vi "get_version_numbering.vi"(11 "local version in":string) -> (0 "resulting string":string, 1 "revision out":i32, 2 "minor out":i32, 3 "mayor out":i32)   [LabVIEW 2010, in "HelioUpdateMH100803.lvclass"]
uses:
  HelioUpdateMH100803.lvclass
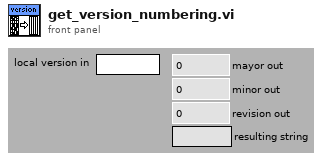
[diagram p1: front panel]
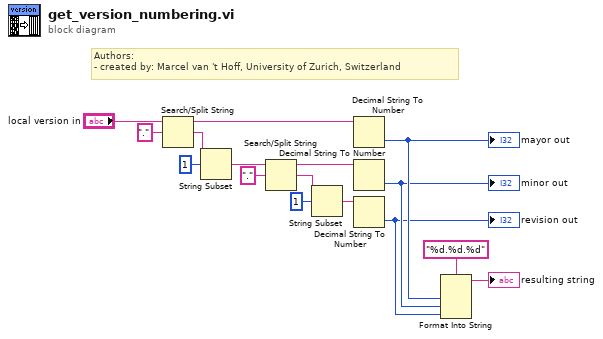
[diagram p0: block diagram]
diagram:
  # "Authors: \n- created by: Marcel van 't Hoff, University of Zurich, Switzerland"
  n1 = Search/Split String(string="local version in", search string/char (-)=".") -> (substring before match=w9:string, match + rest of string=w10:string)  [unwired: 1 in, 1 out]
  n2 = String Subset(string=w10, offset (0)=1) -> (substring=w11:string)  [unwired: 1 in]
  n3 = Search/Split String(string=w11, search string/char (-)=".") -> (substring before match=w15:string, match + rest of string=w13:string)  [unwired: 1 in, 1 out]
  n4 = String Subset(string=w13, offset (0)=1) -> (substring=w16:string)  [unwired: 1 in]
  n5 = Decimal String To Number(string=w9) -> (number=w5:i32)  [unwired: 2 in, 1 out]
  "mayor out" <- w5
  n6 = Decimal String To Number(string=w15) -> (number=w4:i32)  [unwired: 2 in, 1 out]
  "minor out" <- w4
  n7 = Decimal String To Number(string=w16) -> (number=w3:i32)  [unwired: 2 in, 1 out]
  "revision out" <- w3
  n8 = Format Into String(format string="%d.%d.%d", w5, w4, w3) -> (resulting string=→"resulting string":string)  [unwired: 2 in, 1 out]
